vi "Refactored_TipDown.vi"(8 "error in (no error)":errorcluster, 10 "Z Setpoint":dbl, 11 "Application":refnum<k7>) -> (0 "error out":errorcluster, 1 "Y Setpoint":dbl, 2 "X Setpoint":dbl, 3 "Application":refnum<k7>)   [LabVIEW 2016]
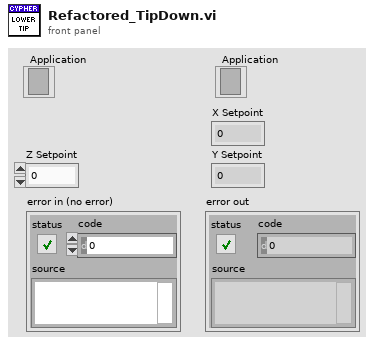
[diagram p1: front panel]
types:
  T1 = cluster{"setpoint":string, "pgain":string, "igain":string, "sgain":string}
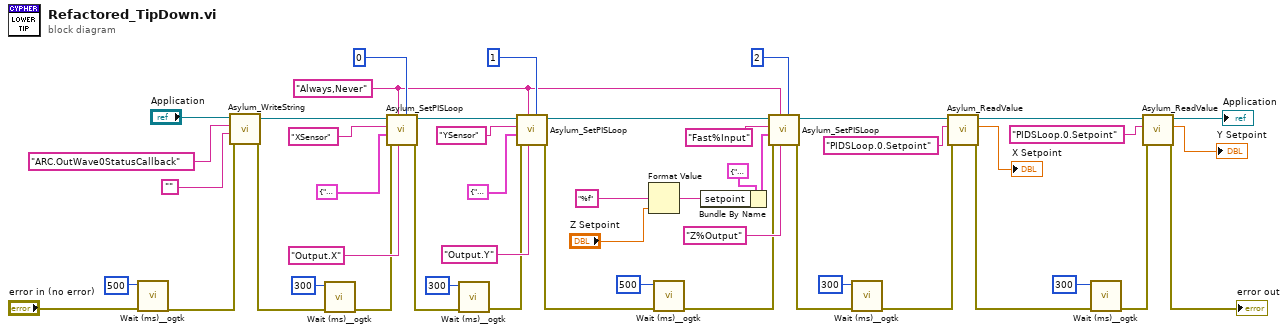
[diagram p0: block diagram]
diagram:
  w31 = "Always,Never" ("eventString")
  n1 = call <userlib>:"Wait (ms)__ogtk.vi"("error in (no error)"="error in (no error)", "milliseconds to wait"=u32 500) -> ("error out"=w18:errorcluster)  [unwired: 8 in, 1 out]
  n2 = call "Asylum_WriteString.vi"("error in (no error)"=w18, "valueString"="", "parameterName"="ARC.OutWave0StatusCallback", "Application"="Application") -> ("error out"=w17:errorcluster, "Application"=w44:refnum<k7>)  [unwired: 6 in]
  n3 = call <userlib>:"Wait (ms)__ogtk.vi"("error in (no error)"=w17, "milliseconds to wait"=u32 300) -> ("error out"=w16:errorcluster)  [unwired: 8 in, 1 out]
  n4 = call "Asylum_SetPISLoop.vi"("whichLoop"=0, "outChannelString"="Output.X", "eventString"=w31, "error in (no error)"=w16, "PIS Controls"=T1 {"setpoint"="NAN", "pgain"="0", "igain"="-63096", "sgain"="0"}, "inChannelString"="XSensor", "Application"=w44) -> ("error out"=w15:errorcluster, "Application"=w39:refnum<k7>)  [unwired: 3 in]
  n5 = call <userlib>:"Wait (ms)__ogtk.vi"("error in (no error)"=w15, "milliseconds to wait"=u32 300) -> ("error out"=w14:errorcluster)  [unwired: 8 in, 1 out]
  n6 = call "Asylum_SetPISLoop.vi"("whichLoop"=1, "outChannelString"="Output.Y", "eventString"=w31, "error in (no error)"=w14, "PIS Controls"=T1 {"setpoint"="NAN", "pgain"="0", "igain"="-63096", "sgain"="0"}, "inChannelString"="YSensor", "Application"=w39) -> ("error out"=w13:errorcluster, "Application"=w30:refnum<k7>)  [unwired: 3 in]
  n7 = Format Value(format string="%f", value (0)="Z Setpoint") -> (output string=w27:string)  [unwired: 1 in]
  n8 = call <userlib>:"Wait (ms)__ogtk.vi"("error in (no error)"=w13, "milliseconds to wait"=u32 500) -> ("error out"=w11:errorcluster)  [unwired: 8 in, 1 out]
  n9 = Bundle By Name(cluster=T1 {"setpoint"="0", "pgain"="0", "igain"="1000", "sgain"="0"} ("PIS Controls"), "setpoint"=w27) -> (w24:T1)
  n10 = call "Asylum_SetPISLoop.vi"("whichLoop"=2, "outChannelString"="Z%Output", "eventString"=w31, "error in (no error)"=w11, "PIS Controls"=w24, "inChannelString"="Fast%Input", "Application"=w30) -> ("error out"=w12:errorcluster, "Application"=w22:refnum<k7>)  [unwired: 3 in]
  n11 = call <userlib>:"Wait (ms)__ogtk.vi"("error in (no error)"=w12, "milliseconds to wait"=u32 300) -> ("error out"=w10:errorcluster)  [unwired: 8 in, 1 out]
  n12 = call "Asylum_ReadValue.vi"("error in (no error)"=w10, "Value"="PIDSLoop.0.Setpoint", "Application"=w22) -> ("error out"=w8:errorcluster, "Value"=→"X Setpoint":dbl, "Application"=w6:refnum<k7>)  [unwired: 6 in]
  n13 = call <userlib>:"Wait (ms)__ogtk.vi"("error in (no error)"=w8, "milliseconds to wait"=u32 300) -> ("error out"=w7:errorcluster)  [unwired: 8 in, 1 out]
  n14 = call "Asylum_ReadValue.vi"("error in (no error)"=w7, "Value"="PIDSLoop.0.Setpoint", "Application"=w6) -> ("error out"=→"error out":errorcluster, "Value"=→"Y Setpoint":dbl, "Application"=→"Application":refnum<k7>)  [unwired: 6 in]
